vi "Execute Command.vi"(8 "error in (no error)":errorcluster, 10 "UI Initialize in":refnum<class "UI Initialize.lvclass">, 11 "User Interface References":T1={"This VI"=refnum, "User Interace Plugin"=refnum, "UI Picture Container References"={"Header Image"=refnum, "Footer Image"=refnum}, "Sliding Menu XControl"=refnum, "Menu Container"=refnum, "UI Configuration Information"={"Space Between Buttons"=3, "Number of Buttons to Show"=6, "Header Image"=path "Images/Blue Background.bmp", "Footer Image"=path "Images/Blue Background.bmp"}, "Header Text"=refnum}) -> (0 "error out":errorcluster, 1 "Stop?":bool, 2 "UI Initialize out":refnum<class "UI Initialize.lvclass">, 3 "User Interface References Out":T1={"This VI"=refnum, "User Interace Plugin"=refnum, "UI Picture Container References"={"Header Image"=refnum, "Footer Image"=refnum}, "Sliding Menu XControl"=refnum, "Menu Container"=refnum, "UI Configuration Information"={"Space Between Buttons"=3, "Number of Buttons to Show"=6, "Header Image"=path "Images/Blue Background.bmp", "Footer Image"=path "Images/Blue Background.bmp"}, "Header Text"=refnum})   [LabVIEW 2011, in "UI Initialize.lvclass"]
uses:
  UI Initialize.lvclass
  Main Type Definitions/User Interface Type Definitions.ctl
  Main Type Definitions/UI Picture Containers.ctl
  Sliding Menu/Sliding Menu Library/Sliding Menu xControl/Sliding Menu XControl.xctl
  UI Control Definitions/UI Configuration Information.ctl
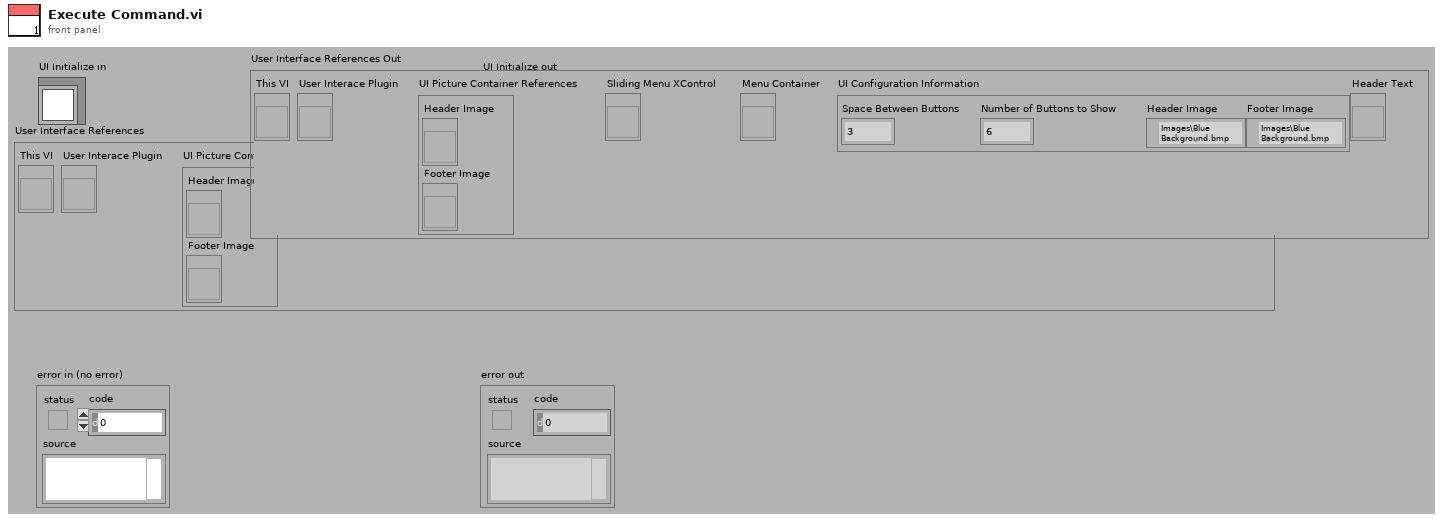
[diagram p1: front panel]
types:
  T1 = typedef "User Interface Type Definitions.ctl" = cluster{"This VI":refnum<vi>, "User Interace Plugin":refnum<vi>, "UI Picture Container References":T2, "Sliding Menu XControl":refnum<vi>, "Menu Container":refnum<vi>, "UI Configuration Information":T3, "Header Text":refnum<vi>}
  T2 = typedef "UI Picture Containers.ctl" = cluster{"Header Image":refnum<vi>, "Footer Image":refnum<vi>}
  T3 = typedef "UI Configuration Information.ctl" = cluster{"Space Between Buttons":i32, "Number of Buttons to Show":i32, "Header Image":path, "Footer Image":path}
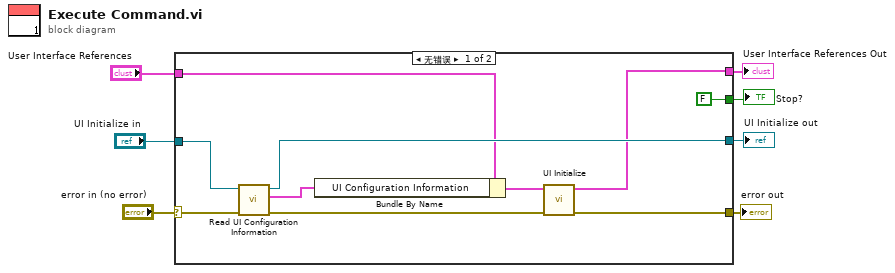
[diagram p0: block diagram]
diagram:
  n1 = case shown="无错误" "error in (no error)" {
    selector: "error in (no error)" -> [w12 w19]
    tunnel: [w17 w19] -> w7
    tunnel: "UI Initialize in" -> [w16 w20]
    tunnel: [w14 w20] -> w5
    tunnel: "User Interface References" -> [w10 w18]
    tunnel: [w11 w18] -> w2
    tunnel: [FALSE ("Stop?") _] -> w1
    frame No Error {
      n2 = call "Read UI Configuration Information.vi"("error in (no error)"=w12, "UI Initialize in"=w16) -> ("error out"=w15:errorcluster, "UI Configuration Information"=w13:T3, "UI Initialize out"=w14:refnum<class "UI Initialize.lvclass">)  [unwired: 7 in]
      n3 = Bundle By Name(cluster=w10, "UI Configuration Information"=w13) -> (w9:T1)
      n4 = call "UI Initialize.vi"("error in (no error)"=w15, "User Interface References"=w9) -> ("error out"=w17:errorcluster, "User Interface References Out"=w11:T1)  [unwired: 8 in]
    }
    frame Error {
    }
  }
  "error out" <- w7
  "UI Initialize out" <- w5
  "Stop?" <- w1
  "User Interface References Out" <- w2
